vi "Read MotionData.vi"(8 "error in (no error)":errorcluster, 10 "ReadSize":u32, 11 "AODAcq in":refnum<class "AODAcq.lvclass">) -> (0 "error out":errorcluster, 2 "MotionData":waveform(i32)[](array[waveform]), 3 "AODAcq out":refnum<class "AODAcq.lvclass">)   [LabVIEW 2011, in "AODAcq.lvclass"]
uses:
  AODAcq.lvclass
  AODAcq.lvclass/AODAcq.ctl
  <instrlib>/niHWS/nihws.llb/niHWS Set Wfm DBL Attribute ID.ctl
  <vilib>/Utility/error.llb/Error Cluster From Error Code.vi
  <vilib>/rvi/errors/niLvFpgaAdjustHostInterfaceError.vi
  <instrlib>/niHWS/nihws.llb/niHWS Write Analog I32.vi
  <vilib>/rvi/interface/nirviMethod/nirviMethod.xnode
  FPGA_Control/AODRef.ctl
  FPGA_Control/FPGA Bitfiles/AODControl_FPGATarget_5751Acquire_F1CF9257.lvbitx
  FPGA_Control/AOD Control (FPGA).vi
  <vilib>/FPGAPlugInAG/PXIe-7965R/niLvFpga_ReadFifo_PXIe-7965R.vi
  <vilib>/rvi/errors/niLvFpgaMergeErrorWithErrorCode.vi
panel:
  out "Samples":i32
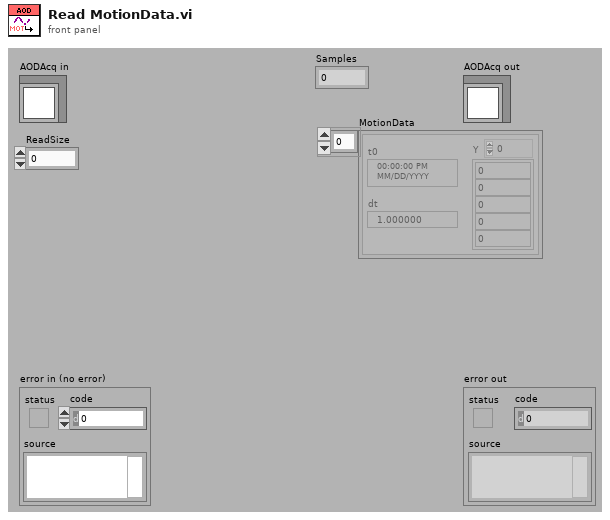
[diagram p1: front panel]
types:
  T1 = typedef "AODRef.ctl" = refnum<k20>
  T2 = typedef "niHWS Set Wfm DBL Attribute ID.ctl" = u32
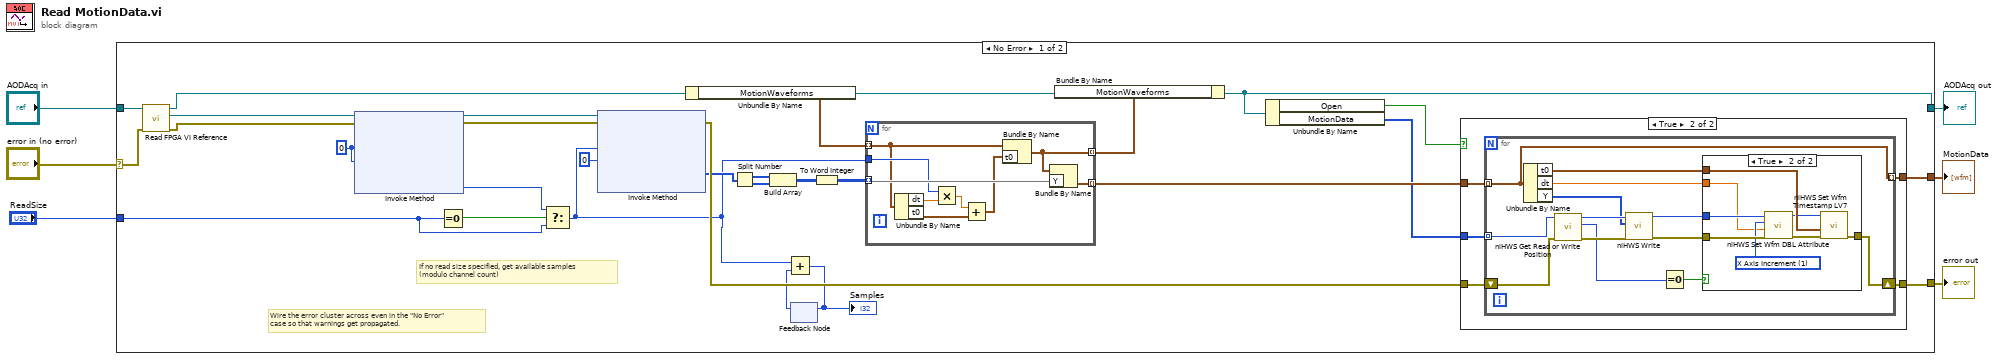
[diagram p0: block diagram]
diagram:
  n1 = case shown="No Error" "error in (no error)" {
    selector: "error in (no error)" -> [w29 w75]
    tunnel: [w20 w75] -> w5
    tunnel: [w24 w74] -> w3
    tunnel: "AODAcq in" -> [w35 w74]
    tunnel: "ReadSize" -> [w8 _]
    tunnel: [w19 _] -> w1
    frame No Error {
      w34 = u32 0 ("Number of Elements")
      # "If no read size specified, get available samples \n(modulo channel count)"
      # "Wire the error cluster across even in the \"No Error\"\ncase so that warnings get propagated."
      n2 = call-dynamic "Read FPGA VI Reference.vi"("error in (no error)"=w29, "AODAcq in"=w35) -> ("error out"=w9:errorcluster, "FPGA VI Reference"=w10:T1, "AODAcq out"=w27:refnum<class "AODAcq.lvclass">)  [unwired: 7 in]
      n3 = xnode "Invoke Method"("FPGA VI Reference In"=w10, "error in"=w9, "Number of Elements"=w34, "Timeout (ms)"=w34) -> ("FPGA VI Reference Out"=w32:T1, "error out"=w31:errorcluster, "Elements Remaining"=w7:u32)  [unwired: 1 out]
      n4 = Equal To 0?(x=w8) -> (x = 0?=w33:bool)
      n5 = Select(t=w7, s=w33, f=w8) -> (s? t:f=w11:u32)
      n6 = xnode "Invoke Method"("FPGA VI Reference In"=w32, "error in"=w31, "Number of Elements"=w11, "Timeout (ms)"=0) -> ("error out"=w21:errorcluster, "Data"=w13:i32[])  [unwired: 2 out]
      n7 = Unbundle By Name(w27) -> ("MotionWaveforms"=w28:waveform(i32)[])
      n8 = Split Number(x=w13) -> (hi(x)=w15:u16[], lo(x)=w16:u16[])
      n9 = Build Array(w15, w16) -> (w14:u16[][])
      n10 = feedback #1() -> (w17:u32)  [unwired: 1 in]
      n11 = Add(x=w11, y=w17) -> (x+y=w18:u32)
      "Samples" <- w18
      n12 = feedback-in #1(w18) -> ()
      n13 = To Word Integer(number=w14) -> (16bit integer=w12:i16[][])
      n14 = for {
        tunnel: w12 -> [w73] mode=indexing
        tunnel: [w72] -> w25 mode=indexing
        tunnel: w28 -> [w67] mode=indexing
        tunnel: w11 -> [w70]
        tunnel: [w65] -> w26 mode=indexing
        n15 = Unbundle By Name(w67) -> ("dt"=w71:dbl, "t0"=w68:timestamp)
        n16 = Multiply(x=w70, y=w71) -> (x*y=w69:dbl)
        n17 = Add(x=w69, y=w68) -> (x+y=w66:timestamp)
        n18 = Bundle By Name(cluster=w67, "t0"=w66) -> (w65:waveform(i32))
        n19 = Bundle By Name(cluster=w65, "Y"=w73) -> (w72:waveform(i32))
      }
      n20 = Bundle By Name(cluster=w27, "MotionWaveforms"=w26) -> (w24:refnum<class "AODAcq.lvclass">)
      n21 = Unbundle By Name(w24) -> ("Open"=w23:bool, "MotionData"=w22:u32[])
      n22 = case shown="True" w23 {
        tunnel: w25 -> [w36 w42]
        tunnel: w22 -> [_ w41]
        tunnel: w21 -> [w37 w40]
        tunnel: [w37 w39] -> w20
        tunnel: [w36 w38] -> w19
        frame False {
        }
        frame True {
          n23 = for {
            tunnel: w42 -> [w43] mode=indexing
            tunnel: w41 -> [w47] mode=indexing
            shift-right: [w44] -> w39
            shift-left: w40 -> [w49]
            tunnel: [w43] -> w38 mode=indexing
            n24 = Unbundle By Name(w43) -> ("t0"=w45:timestamp, "dt"=w46:dbl, "Y"=w48:i32[])
            n25 = call <instrlib>:"niHWS Get Read or Write Position.vi"("waveform reference in"=w47, "error in (no error)"=w49) -> ("waveform reference out"=w54:u32, "position"=w51:u32, "error out"=w53:errorcluster)  [unwired: 6 out]
            n26 = call-poly <instrlib>:"niHWS Write.vi"("error in (no error)"=w53, "data"=w48, "waveform reference in"=w54) -> ("error out"=w52:errorcluster, "waveform reference out"=w55:u32)  [unwired: 7 in]
            n27 = Equal To 0?(x=w51) -> (x = 0?=w50:bool)
            n28 = case shown="True" w50 {
              tunnel: w45 -> [_ w63]
              tunnel: [w56 w62] -> w44
              tunnel: w52 -> [w56 w60]
              tunnel: w55 -> [_ w59]
              tunnel: w46 -> [_ w57]
              frame False {
              }
              frame True {
                w58 = T2 1 items=["X Axis Start"=0, "X Axis Increment"=1, "Y Axis Minimum"=3, "Y Axis Maximum"=4] ("Attribute ID")
                n29 = call <instrlib>:"niHWS Set Wfm DBL Attribute.vi"("error in (no error)"=w60, "attribute value"=w57, "attribute ID"=w58, "waveform reference in"=w59) -> ("error out"=w64:errorcluster, "waveform reference out"=w61:u32)  [unwired: 6 out]
                n30 = call <instrlib>:"niHWS Set Wfm Timestamp LV7.vi"("error in (no error)"=w64, "waveform timestamp"=w63, "waveform reference in"=w61) -> ("error out"=w62:errorcluster)  [unwired: 8 out]
              }
            }
          }
        }
      }
    }
    frame Error {
    }
  }
  "error out" <- w5
  "AODAcq out" <- w3
  "MotionData" <- w1
